vi "fillnumber.vi"(9 "map":i8[][][](array[numeric]), 10 "size":i32, 11 "layers":i32) -> (3 "Array out":i8[][][](array[numeric]))   [LabVIEW 2025]
uses:
  <vilib>/Utility/file.llb/Write Delimited Spreadsheet (I64).vi
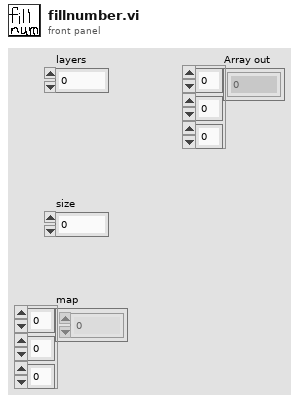
[diagram p1: front panel]
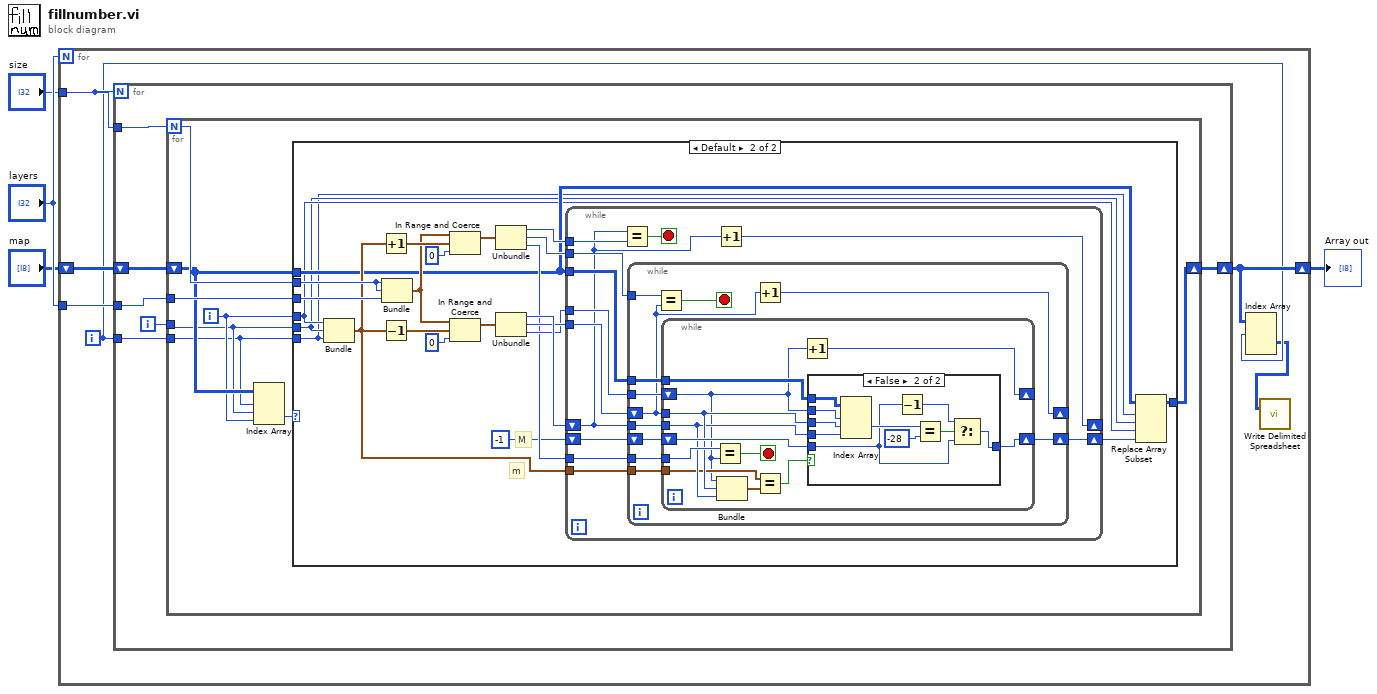
[diagram p0: block diagram]
diagram:
  n1 = for {
    N: "layers" -> [_]
    tunnel: "size" -> [w9]
    tunnel: "layers" -> [w8]
    shift-right: [w7] -> w4
    shift-left: "map" -> [w10]
    i -> [w6]
    n2 = for {
      N: w9 -> [_]
      tunnel: w9 -> [w15]
      tunnel: w6 -> [w14]
      tunnel: w8 -> [w12]
      shift-right: [w11] -> w7
      shift-left: w10 -> [w16]
      i -> [w13]
      n3 = for {
        N: w15 -> [w24]
        tunnel: w14 -> [w18]
        tunnel: w13 -> [w19]
        tunnel: w12 -> [w23]
        shift-right: [w22] -> w11
        shift-left: w16 -> [w21]
        i -> [w20]
        n4 = Index Array(array=w21, index (dim 0)=w18, index (dim 1)=w19, index (dim 2)=w20) -> (element=w17:i8)
        n5 = case shown="Default" w17 {
          tunnel: w24 -> [_ w48]
          tunnel: w23 -> [_ w47]
          tunnel: [w25 w32] -> w22
          tunnel: w21 -> [w25 w29]
          tunnel: w20 -> [_ w28]
          tunnel: w19 -> [_ w27]
          tunnel: w18 -> [_ w26]
          frame -30, -28, 0 {
          }
          frame Default {
            # "m"
            # "M"
            n6 = Bundle(w28, w27, w26) -> (w30:cluster{i32, i32, i32})  [unwired: 1 in]
            n7 = Increment(x=w30) -> (x+1=w46:cluster{i32, i32, i32})
            n8 = Decrement(x=w30) -> (x-1=w43:cluster{i32, i32, i32})
            n9 = Bundle(w48, w48, "layers"=w47) -> (w42:cluster{i32, i32, "layers":i32})  [unwired: 1 in]
            n10 = In Range and Coerce(upper limit=w42, x=w46, lower limit=0) -> (coerced(x)=w33:cluster{i32, i32, "layers":i32})  [unwired: 1 out]
            n11 = In Range and Coerce(upper limit=w42, x=w43, lower limit=0) -> (coerced(x)=w34:cluster{i32, i32, "layers":i32})  [unwired: 1 out]
            n12 = Unbundle(w33) -> (w40:i32, w39:i32, "layers"=w36:i32)
            n13 = Unbundle(w34) -> (w41:i32, w38:i32, "layers"=w37:i32)
            n14 = while {
              shift-right: [w60] -> _
              shift-left: w41 -> [w52]
              tunnel: w40 -> [w59]
              tunnel: w39 -> [w57]
              tunnel: w38 -> [w56]
              tunnel: w37 -> [w55]
              tunnel: w36 -> [w54]
              tunnel: w29 -> [w53]
              shift-right: [w50] -> w31
              shift-left: i8 -1 -> [w51]
              tunnel: w30 -> [w49]
              stop <- w58 stop-if-true
              n15 = Equal?(x=w52, y=w59) -> (x = y?=w58:bool)
              n16 = while {
                tunnel: w57 -> [w70]
                shift-right: [w61] -> _
                shift-left: w56 -> [w66]
                tunnel: w55 -> [w69]
                tunnel: w54 -> [w68]
                tunnel: w53 -> [w67]
                tunnel: w52 -> [w65]
                shift-right: [w63] -> w50
                shift-left: w51 -> [w64]
                tunnel: w49 -> [w62]
                stop <- w71 stop-if-true
                n17 = Equal?(x=w70, y=w66) -> (x = y?=w71:bool)
                n18 = while {
                  shift-right: [w72] -> _
                  shift-left: w69 -> [w73]
                  tunnel: w68 -> [w82]
                  tunnel: w67 -> [w81]
                  tunnel: w66 -> [w78]
                  tunnel: w65 -> [w77]
                  shift-right: [w80] -> w63
                  shift-left: w64 -> [w79]
                  tunnel: w62 -> [w76]
                  stop <- w83 stop-if-true
                  n19 = Equal?(x=w82, y=w73) -> (x = y?=w83:bool)
                  n20 = Bundle("layers"=w73, w78, w77) -> (w75:cluster{"layers":i32, i32, i32})  [unwired: 1 in]
                  n21 = Equal?(x=w76, y=w75) -> (x = y?=w74:bool)
                  n22 = Increment(x=w73) -> (x+1=w72:i32)
                  n23 = case shown="False" w74 {
                    tunnel: w81 -> [_ w94]
                    tunnel: w73 -> [_ w93]
                    tunnel: w78 -> [_ w92]
                    tunnel: w77 -> [_ w91]
                    tunnel: [w84 w89] -> w80
                    tunnel: w79 -> [w84 w87]
                    frame True {
                    }
                    frame False {
                      n24 = Index Array(array=w94, index (dim 0)=w93, index (dim 1)=w92, index (dim 2)=w91) -> (element=w88:i8)
                      n25 = Decrement(x=w87) -> (x-1=w86:i8)
                      n26 = Equal?(x=w88, y=i8 -28) -> (x = y?=w85:bool)
                      n27 = Select(t=w86, s=w85, f=w87) -> (s? t:f=w89:i8)
                    }
                  }
                }
                n28 = Increment(x=w66) -> (x+1=w61:i32)
              }
              n29 = Increment(x=w52) -> (x+1=w60:i32)
            }
            n30 = Replace Array Subset(array=w29, new element=w31, index (dim 0)=w26, index (dim 1)=w27, index (dim 2)=w28) -> (w32:i8[][][])
          }
        }
      }
    }
    n31 = Index Array(array=w7, index (dim 0)=w6) -> (element=w5:i8[][])  [unwired: 2 in]
    n32 = call-poly <vilib>:"Write Delimited Spreadsheet.vi"("2D data"=w5) -> ()  [unwired: 13 in, 2 out]
  }
  "Array out" <- w4
